vi "is visible to load.vi"(8 "error in":errorcluster, 11 "TEST EDITOR in":refnum<class "TEST EDITOR.lvclass">) -> (0 "error out":errorcluster, 2 "visible":bool, 3 "TEST EDITOR out":refnum<class "TEST EDITOR.lvclass">)   [LabVIEW 2013, in "configuration tests.lvlib" / "TEST EDITOR.lvclass"]
doc: "Determines whether a node should be visible when generating right click menus. By default, any abstract node is not visible."
uses:
  TEST EDITOR.lvclass
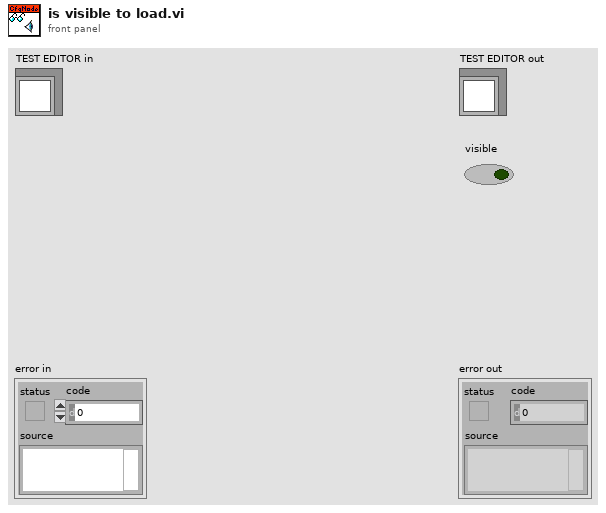
[diagram p1: front panel]
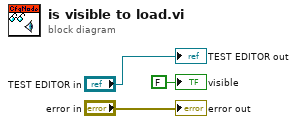
[diagram p0: block diagram]
diagram:
  "error out" <- "error in"
  "TEST EDITOR out" <- "TEST EDITOR in"
  "visible" <- FALSE ("visible")
